vi "Write IFDs.vi"(8 "error in (no error)":errorcluster, 11 "TIFF in":refnum<class "TIFF.lvclass">) -> (0 "error out":errorcluster, 3 "TIFF out":refnum<class "TIFF.lvclass">)   [LabVIEW 2018, in "BinaryTIFF.lvlib" / "TIFF.lvclass"]
uses:
  TIFF.lvclass
  TIFF.lvclass/TIFF.ctl
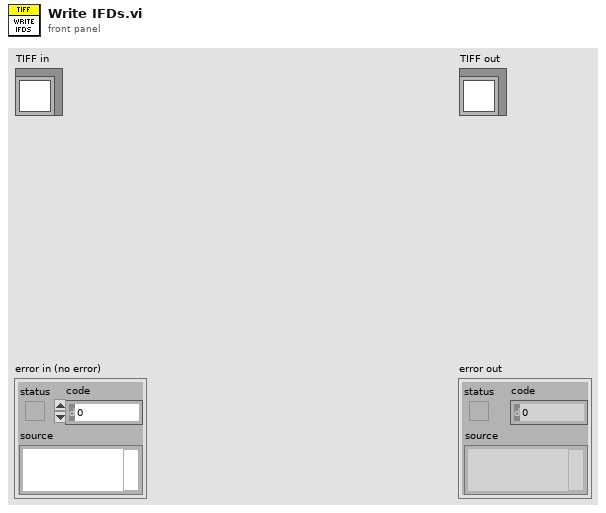
[diagram p1: front panel]
types:
  T1 = enum16{"big-endian, network order", "native, host order", "little-endian"}
  T2 = cluster{"Offset":u64, "Number of Entries":u64, "IFD Entries":cluster{"Tag":u16, "Data Type":u16, "Number of Elements":u64, "Data":variant}[]}[]
  T3 = cluster{"Tag":u16, "Data Type":u16, "Number of Elements":u64, "Data":variant}[]
  T4 = cluster{"Offset":u64, "Number of Entries":u64, "IFD Entries":cluster{"Tag":u16, "Data Type":u16, "Number of Elements":u64, "Data":variant}[]}
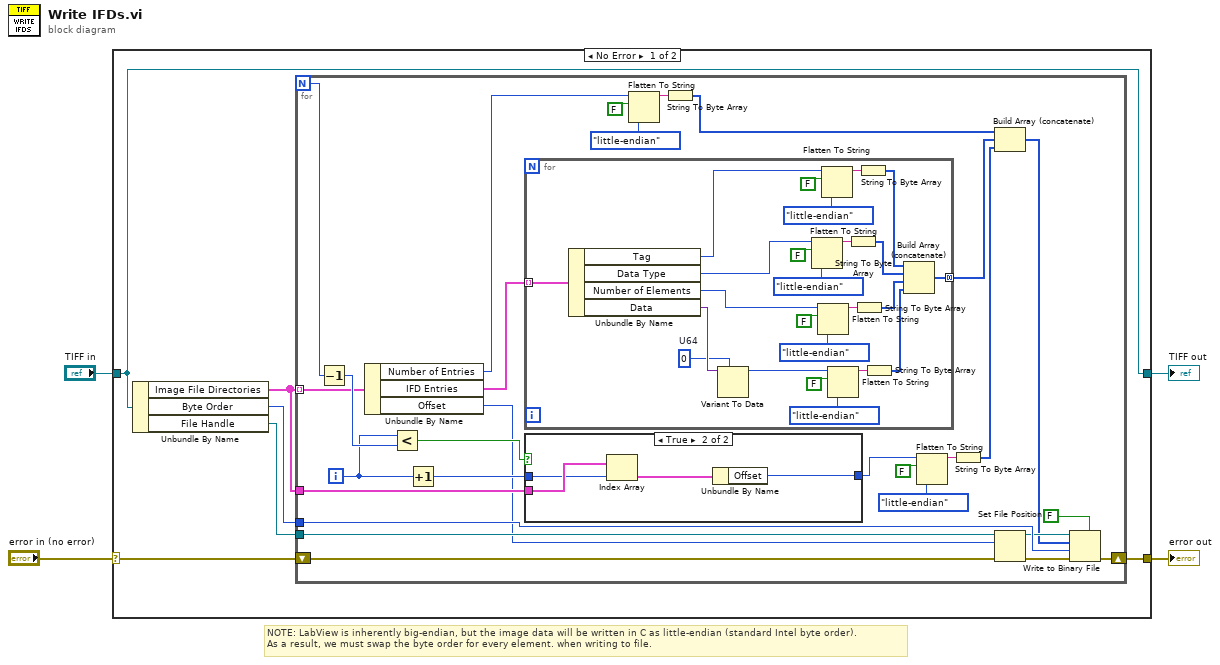
[diagram p0: block diagram]
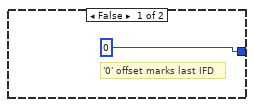
[diagram p2: hidden frame]
diagram:
  # "NOTE: LabView is inherently big-endian, but the image data will be written in C as little-endian (standard Intel byte order).\nAs a result, we must swap the byte order for every element. when writing to file."
  n1 = case shown="No Error" "error in (no error)" {
    selector: "error in (no error)" -> [w8 w69]
    tunnel: [w7 w69] -> w3
    tunnel: [w10 w68] -> w1
    tunnel: "TIFF in" -> [w10 w68]
    frame No Error {
      n2 = Unbundle By Name(w10) -> ("Image File Directories"=w9:T2, "Byte Order"=w5:T1, "File Handle"=w6:refnum<file>)
      n3 = for {
        N -> [w37]
        tunnel: w9 -> [w34] mode=indexing
        tunnel: w9 -> [w38]
        tunnel: w6 -> [w31]
        tunnel: w5 -> [w30]
        shift-right: [w26] -> w7
        shift-left: w8 -> [w27]
        i -> [w35]
        n4 = Decrement(x=w37) -> (x-1=w36:i32)
        n5 = Unbundle By Name(w34) -> ("Number of Entries"=w12:u64, "IFD Entries"=w33:T3, "Offset"=w11:u64)
        n6 = Less?(x=w35, y=w36) -> (x < y?=w22:bool)
        n7 = Increment(x=w35) -> (x+1=w23:i32)
        n8 = for {
          tunnel: w33 -> [w67] mode=indexing
          tunnel: [w66] -> w32 mode=concatenating
          w64 = u64 0  # U64
          n9 = Unbundle By Name(w67) -> ("Tag"=w60:u16, "Data Type"=w50:u16, "Number of Elements"=w55:u64, "Data"=w65:variant)
          n10 = Variant To Data(type=w64, Variant=w65) -> (data=w44:u64)  [unwired: 1 in, 1 out]
          n11 = Flatten To String(anything=w50, prepend array or string size? (T)=FALSE, byte order (0:big-endian, network order)=T1."little-endian") -> (data string=w52:string)  [unwired: 1 in, 2 out]
          n12 = Flatten To String(anything=w55, prepend array or string size? (T)=FALSE, byte order (0:big-endian, network order)=T1."little-endian") -> (data string=w57:string)  [unwired: 1 in, 2 out]
          n13 = Flatten To String(anything=w60, prepend array or string size? (T)=FALSE, byte order (0:big-endian, network order)=T1."little-endian") -> (data string=w62:string)  [unwired: 1 in, 2 out]
          n14 = Flatten To String(anything=w44, prepend array or string size? (T)=FALSE, byte order (0:big-endian, network order)=T1."little-endian") -> (data string=w47:string)  [unwired: 1 in, 2 out]
          n15 = String To Byte Array(string=w52) -> (unsigned byte array=w49:u8[])
          n16 = String To Byte Array(string=w57) -> (unsigned byte array=w54:u8[])
          n17 = String To Byte Array(string=w62) -> (unsigned byte array=w59:u8[])
          n18 = String To Byte Array(string=w47) -> (unsigned byte array=w45:u8[])
          n19 = Build Array (concatenate)(w59, w49, w54, w45) -> (w66:u8[])
        }
        n20 = case shown="True" w22 {
          tunnel: w38 -> [_ w43]
          tunnel: w23 -> [_ w42]
          tunnel: [u64 0 ("Offset") w40] -> w20
          frame False {
            # "'0' offset marks last IFD"
          }
          frame True {
            n21 = Index Array(array=w43, index=w42) -> (element=w41:T4)
            n22 = Unbundle By Name(w41) -> ("Offset"=w40:u64)
          }
        }
        n23 = Flatten To String(anything=w12, prepend array or string size? (T)=FALSE, byte order (0:big-endian, network order)=T1."little-endian") -> (data string=w15:string)  [unwired: 1 in, 2 out]
        n24 = String To Byte Array(string=w15) -> (unsigned byte array=w13:u8[])
        n25 = Flatten To String(anything=w20, prepend array or string size? (T)=FALSE, byte order (0:big-endian, network order)=T1."little-endian") -> (data string=w19:string)  [unwired: 1 in, 2 out]
        n26 = String To Byte Array(string=w19) -> (unsigned byte array=w18:u8[])
        n27 = Build Array (concatenate)(w13, w32, w18) -> (w25:u8[])
        n28 = Set File Position(offset (in bytes) (0)=w11, refnum=w31, error in=w27) -> (refnum out=w28:refnum<file>, error out=w29:errorcluster)  [unwired: 1 in]
        n29 = Write to Binary File(file (use dialog)=w28, data=w25, error in=w29, 5:FALSE ("prepend array or string size? (T)"), 9:w30) -> (error out=w26:errorcluster)  [unwired: 1 in, 2 out]
      }
    }
    frame Error {
    }
  }
  "error out" <- w3
  "TIFF out" <- w1
